vi "Close Connection.vi"(8 "error in (no error)":errorcluster, 11 "mysql in":refnum<class "mysql.lvclass">) -> (0 "error out":errorcluster, 3 "mysql out":refnum<class "mysql.lvclass">)   [LabVIEW 2020, in "mysql.lvlib" / "mysql.lvclass"]
uses:
  mysql.lvclass
  mysql.lvclass/mysql.ctl
  MySql.Data
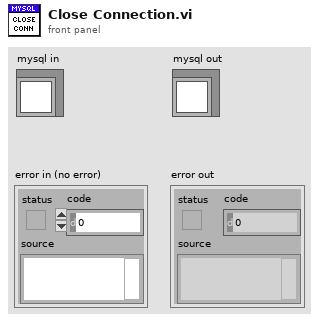
[diagram p1: front panel]
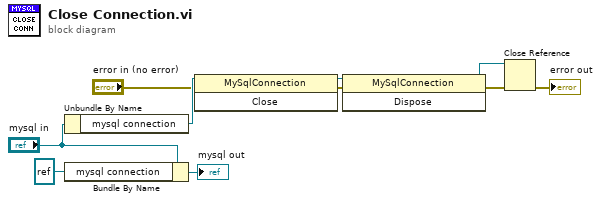
[diagram p0: block diagram]
diagram:
  n1 = Unbundle By Name("mysql in") -> ("mysql connection"=w7:refnum<k24>)
  n2 = Bundle By Name(cluster="mysql in", "mysql connection"=refnum<k24> refnum) -> (→"mysql out":refnum<class "mysql.lvclass">)
  n3 = invoke class="MySqlConnection" method="Close"(reference=w7, error in="error in (no error)") -> (reference out=w10:refnum<k24>, error out=w9:errorcluster)  [unwired: 1 in, 1 out]
  n4 = invoke class="MySqlConnection" method="Dispose"(reference=w10, error in=w9) -> (reference out=w2:refnum<k24>, error out=w8:errorcluster)  [unwired: 1 in, 1 out]
  n5 = Close Reference(reference=w2, error in (no error)=w8) -> (error out=→"error out":errorcluster)
